vi "LithographyDataToVariant.vi"(11 "Lithography Data In":T3(array[cluster])) -> (3 "Lithography Data Out":T2(array[cluster]))   [LabVIEW 2020]
uses:
  <userlib>/LevyLab/Relay Box/Type_defs/Resistor--enum.ctl
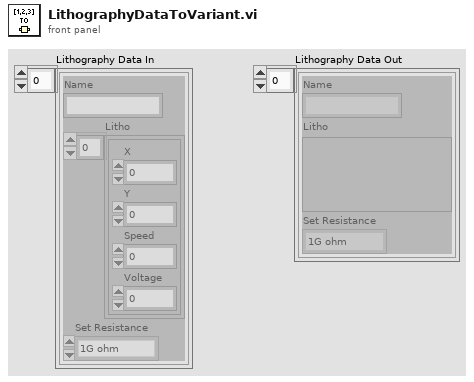
[diagram p1: front panel]
types:
  T1 = typedef "Resistor--enum.ctl" = enum16{"open", "discharge tip", "0 ohms", "100k ohm", "10M ohm", "1G ohm"}
  T2 = cluster{"Name":string, "Litho":variant, "Set Resistance":T1}[]
  T3 = cluster{"Name":string, "Litho":cluster{"X":dbl, "Y":dbl, "Speed":dbl, "Voltage":dbl}[], "Set Resistance":T1}[]
  T4 = cluster{"X":dbl, "Y":dbl, "Speed":dbl, "Voltage":dbl}[]
  T5 = cluster{"Name":string, "Litho":variant, "Set Resistance":T1}
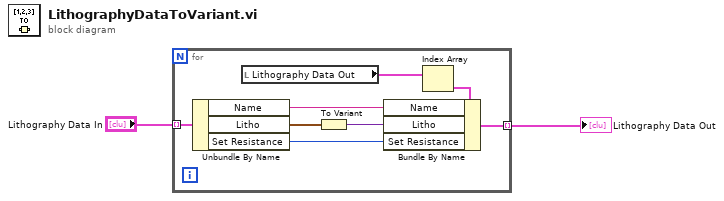
[diagram p0: block diagram]
diagram:
  n1 = for {
    tunnel: "Lithography Data In" -> [w10] mode=indexing
    tunnel: [w3] -> w1 mode=indexing
    n2 = Unbundle By Name(w10) -> ("Name"=w5:string, "Litho"=w9:T4, "Set Resistance"=w4:T1)
    n3 = local read "Lithography Data Out"() -> (w7:T2)
    n4 = To Variant(anything=w9) -> (Variant=w8:variant)
    n5 = Index Array(array=w7) -> (element=w6:T5)  [unwired: 1 in]
    n6 = Bundle By Name(cluster=w6, "Name"=w5, "Litho"=w8, "Set Resistance"=w4) -> (w3:T5)
  }
  "Lithography Data Out" <- w1
